vi "Perform Measurements.vi"(7 "error in":errorcluster, 8 "Measurement Context":refnum<class "Measure Call Context.lvclass">, 9 "Nominal output voltage":dbl, 10 "Reference values":T2) -> (0 "error out":errorcluster, 1 "Measurement Results":T1, 2 "Load out":refnum<k15>, 3 "Source out":refnum<k15>)   [LabVIEW 2021, in "Efficiency And Load Regulation_PMIC.lvlib"]
uses:
  Efficiency And Load Regulation_PMIC.lvlib
  Measurement Results.ctl
  <vilib>/MeasurementLink/MeasurementLink Measurement Server/Measure Call Context/Measure Call Context.lvclass
  <vilib>/MeasurementLink/MeasurementLink Measurement Server/Measure Call Context/Accessor/Is Canceled.vi
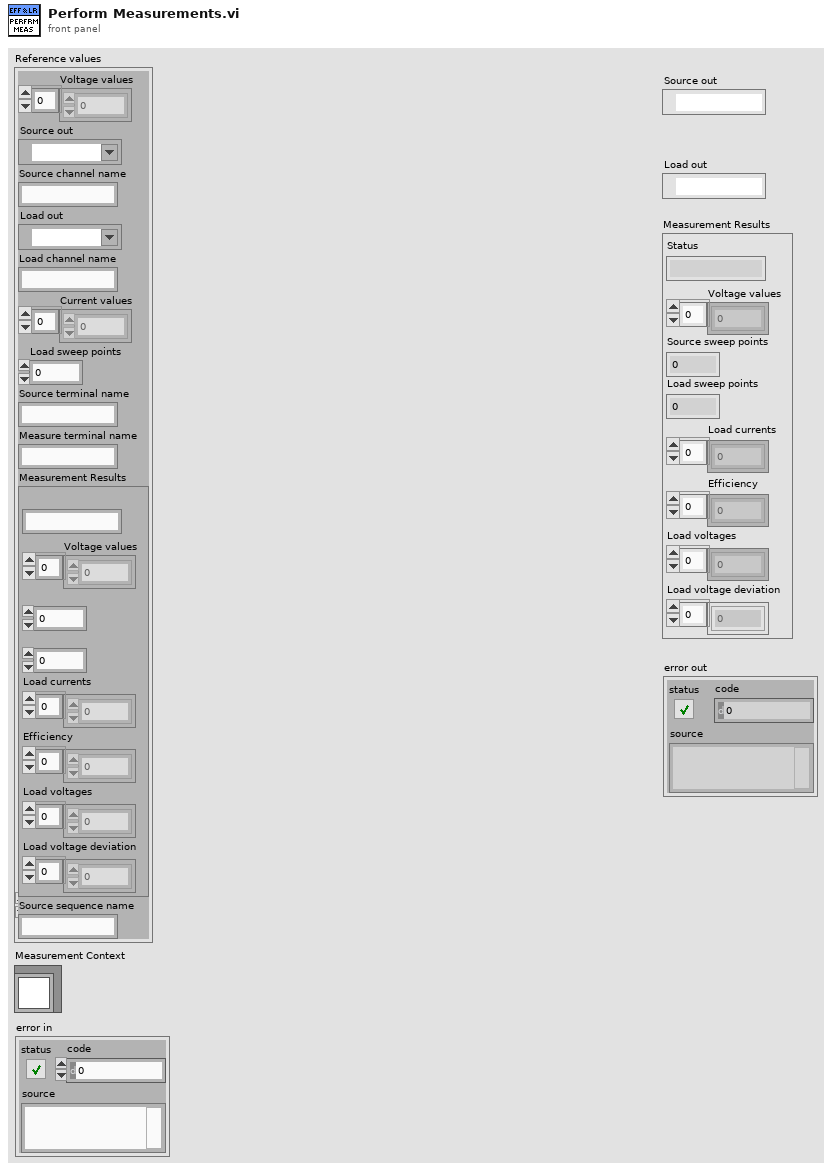
[diagram p1: front panel]
types:
  T1 = typedef "Efficiency And Load Regulation_PMIC.lvlib/Measurement Results.ctl" = cluster{"Status":string, "Voltage values":dbl[], "Source sweep points":i32, "Load sweep points":i32, "Load currents":dbl[], "Efficiency":dbl[], "Load voltages":dbl[], "Load voltage deviation":dbl[]}
  T2 = cluster{"Voltage values":dbl[], "Source out":refnum<k15>, "Source channel name":string, "Load out":refnum<k15>, "Load channel name":string, "Current values":dbl[], "Load sweep points":i32, "Source terminal name":string, "Measure terminal name":string, "Measurement Results":T1, "Source sequence name":string}
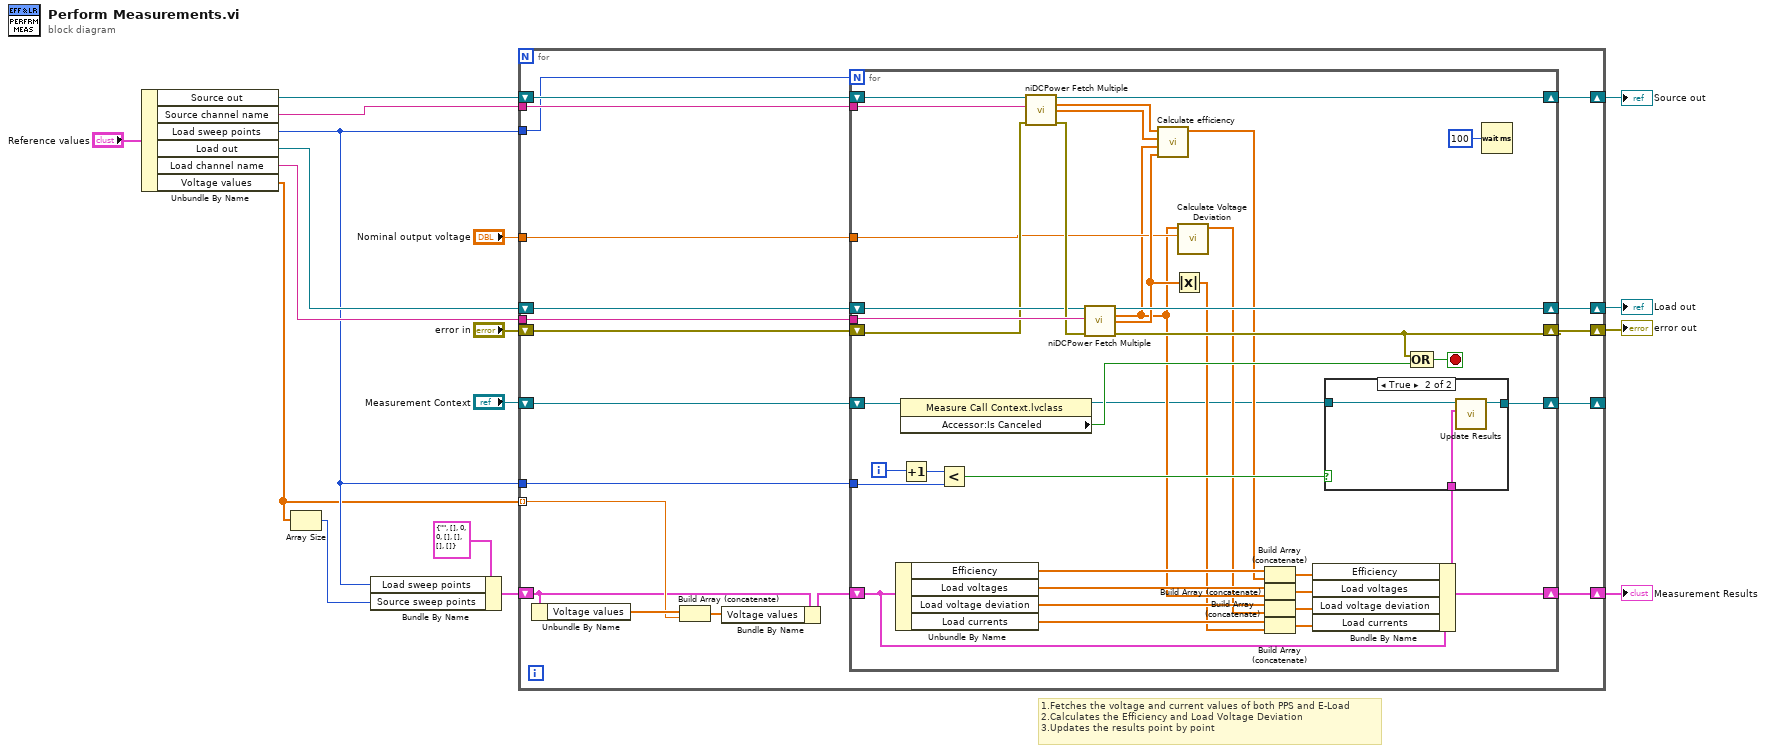
[diagram p0: block diagram]
diagram:
  # "1.Fetches the voltage and current values of both PPS and E-Load\n2.Calculates the Efficiency and Load Voltage Deviation\n3.Updates the results point by point"
  n1 = Unbundle By Name("Reference values") -> ("Source out"=w11:refnum<k15>, "Source channel name"=w10:string, "Load sweep points"=w4:i32, "Load out"=w9:refnum<k15>, "Load channel name"=w8:string, "Voltage values"=w2:dbl[])
  n2 = Array Size(array=w2) -> (size(s)=w1:i32)
  n3 = Bundle By Name(cluster=T1 {"Status"="", "Voltage values"=[], "Source sweep points"=0, "Load sweep points"=0, "Load currents"=[], "Efficiency"=[], "Load voltages"=[], "Load voltage deviation"=[]} ("Measurement Results"), "Load sweep points"=w4, "Source sweep points"=w1) -> (w6:T1)
  n4 = for {
    tunnel: "Nominal output voltage" -> [w32]
    tunnel: w10 -> [w30]
    tunnel: w8 -> [w28]
    tunnel: w4 -> [w27]
    shift-right: [w35] -> w16
    shift-left: "error in" -> [w36]
    shift-right: [w33] -> w14
    shift-left: w11 -> [w31]
    shift-right: [w34] -> w15
    shift-left: w9 -> [w29]
    shift-right: [w25] -> _
    shift-left: "Measurement Context" -> [w26]
    shift-right: [w24] -> w5
    shift-left: w6 -> [w20]
    tunnel: w2 -> [w21] mode=indexing
    tunnel: w4 -> [w23]
    n5 = Unbundle By Name(w20) -> ("Voltage values"=w22:dbl[])
    n6 = Build Array (concatenate)(w22, w21) -> (w18:dbl[])
    n7 = Bundle By Name(cluster=w20, "Voltage values"=w18) -> (w19:T1)
    n8 = for {
      N: w27 -> [_]
      tunnel: w28 -> [w70]
      tunnel: w30 -> [w69]
      shift-right: [w71] -> w34
      shift-left: w29 -> [w67]
      shift-right: [w60] -> w35
      shift-left: w36 -> [w66]
      shift-right: [w72] -> w33
      shift-left: w31 -> [w73]
      tunnel: w32 -> [w62]
      shift-right: [w39] -> w25
      shift-left: w26 -> [w56]
      shift-right: [w42] -> w24
      shift-left: w19 -> [w43]
      tunnel: w23 -> [w38]
      i -> [w58]
      stop <- w41 stop-if-true
      n9 = Unbundle By Name(w43) -> ("Efficiency"=w48:dbl[], "Load voltages"=w49:dbl[], "Load voltage deviation"=w50:dbl[], "Load currents"=w51:dbl[])
      n10 = property class="Measure Call Context.lvclass"(reference=w56) -> (reference out=w40:refnum<class "Measure Call Context.lvclass">, "Accessor:Is Canceled"=w61:bool)  [unwired: 1 in, 1 out]
      n11 = Increment(x=w58) -> (x+1=w59:i32)
      n12 = Less?(x=w59, y=w38) -> (x < y?=w57:bool)
      n13 = call <instrlib>:"niDCPower Fetch Multiple.vi"("instrument handle"=w73, "channel name"=w69, "error in (no error)"=w66) -> ("instrument handle out"=w72:refnum<k15>, "voltage measurements"=w65:dbl[], "current measurements"=w64:dbl[], "error out"=w68:errorcluster)  [unwired: 2 in, 7 out]
      n14 = call <instrlib>:"niDCPower Fetch Multiple.vi"("instrument handle"=w67, "channel name"=w70, "error in (no error)"=w68) -> ("instrument handle out"=w71:refnum<k15>, "voltage measurements"=w46:dbl[], "current measurements"=w63:dbl[], "error out"=w60:errorcluster)  [unwired: 2 in, 7 out]
      n15 = call "Calculate efficiency.vi"("load current measurements"=w63, "load voltage measurements"=w46, "source current measurements"=w64, "source voltage measurements"=w65) -> ("Efficiency(%)"=w47:dbl[])  [unwired: 7 in]
      n16 = Absolute Value(x=w63) -> (abs(x)=w44:dbl[])
      n17 = call "Calculate Voltage Deviation.vi"("Nominal output voltage"=w62, "Voltage measurements"=w46) -> ("Load voltage deviation"=w45:dbl[])  [unwired: 9 in]
      n18 = Build Array (concatenate)(w48, w47) -> (w52:dbl[])
      n19 = Build Array (concatenate)(w49, w46) -> (w53:dbl[])
      n20 = Build Array (concatenate)(w50, w45) -> (w54:dbl[])
      n21 = Build Array (concatenate)(w51, w44) -> (w55:dbl[])
      n22 = Bundle By Name(cluster=w43, "Efficiency"=w52, "Load voltages"=w53, "Load voltage deviation"=w54, "Load currents"=w55) -> (w42:T1)
      n23 = case shown="True" w57 {
        tunnel: w42 -> [_ w77]
        tunnel: w40 -> [w74 w76]
        tunnel: [w74 w75] -> w39
        frame False {
        }
        frame True {
          n24 = call <vilib>:"Update Results.vi"("measurement results"=w77, "measure call context in"=w76) -> ("measure call context out"=w75:refnum<class "Measure Call Context.lvclass">)  [unwired: 8 in, 1 out]
        }
      }
      n25 = Compound Arithmetic op=OR(w60, w61) -> (w41:bool)
      n26 = Wait (ms)(milliseconds to wait=u32 100) -> ()  [unwired: 1 out]
    }
  }
  "error out" <- w16
  "Load out" <- w15
  "Source out" <- w14
  "Measurement Results" <- w5
